vi "Cal Mic Sensitivity.vi"(0 "Device":string) -> (8 "Sens out":dbl)   [LabVIEW 2020]
uses:
  Sub VIs/CalMic-Params.ctl
  <vilib>/DAQmx/read.llb/DAQmx Read (Analog 1D DBL 1Chan NSamp).vi
  <vilib>/Analysis/4window.llb/Hamming Window (DBL).vi
  <vilib>/Analysis/5stat.llb/RMS (DBL).vi
  26d49422-8282-4cac-89f2-fadff3ad3e6e.vi
  d476ff2c-f51a-459e-9784-94b5c1fe9eba.vi
  15152fcf-90b8-4f6a-bf53-2f36ac7739d4.vi
  35692ca8-84b5-411b-8b71-ad00e1a5d34d.vi
  c40c26ba-0181-4530-a77b-ff5f65ea09db.vi
  05361e6f-4f95-456f-9b20-3cc06ed979b3.vi
  d7286415-6cbf-4582-be6d-b454bdd6b62e.vi
  bff657e4-377c-489f-b970-c3d29121513a.vi
  4f9c2216-a235-4407-9711-f98c08391440.vi
  <vilib>/Analysis/baseanly.llb/Mean.vi
  <vilib>/Analysis/baseanly.llb/Mean (DBL).vi
  <vilib>/Analysis/4window.llb/AllCosWindow (DBL).vi
  <vilib>/DAQmx/miscellaneous.llb/DAQmx Fill In Error Info.vi
  epl-vi-lib/Utility VIs/Math VIs/FFT x(t) to dB,Degrees (1D).vi
  <vilib>/Analysis/NI_AALPro.lvlib
  epl-vi-lib/PXI DAQ VIs/TDT VIs/TDT-Signal Bank Action.ctl
panel:
  in  "mV/Pa":dbl=-inf caption="Mic Sens (mV/Pa)"
  in  "Mic Sens (dB V/SPL) in":dbl=-inf
  in  "START":bool
  in  "Sens":dbl=-inf caption="Mic Sens (dB V/SPL)"
  in  "Duration (s)":dbl=1.0
  in  "Sampling Rate (Hz)":dbl=20000.0
  in  "Level (dB SPL)":dbl=124.0 caption="Pistonphone Output\n(dB SPL)" format="%.2f"
  in  "Gain (dB)":dbl=2.0
  out "Magnitude Graph":T1(graph)
  out "Waveform Graph":dbl[](graph)
  in  "finished":errorcluster
  out "Calibration Log":string[][](table)
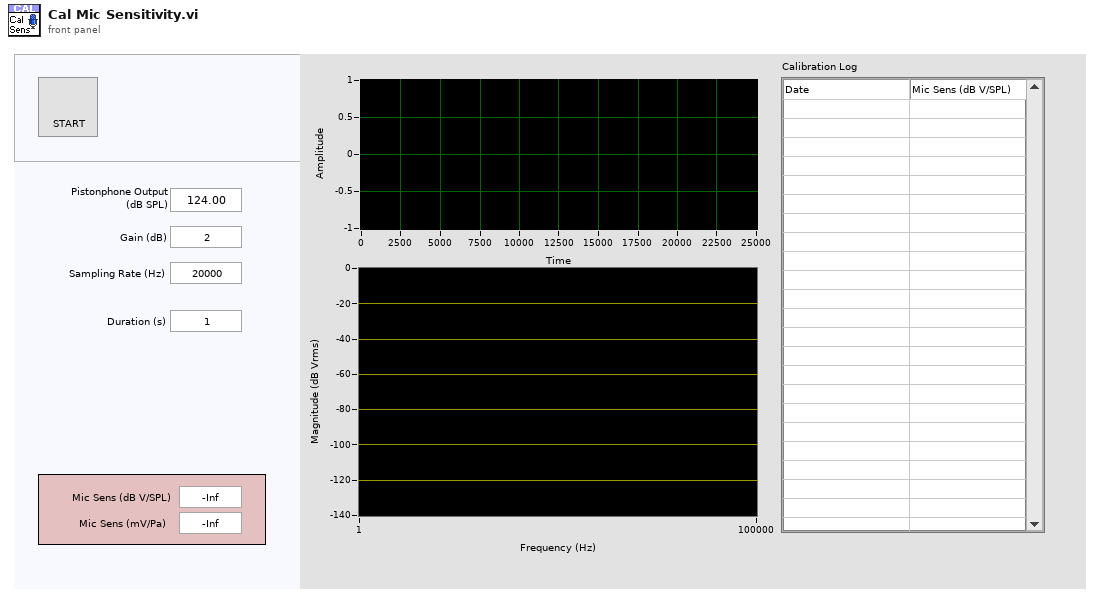
[diagram p1: front panel]
types:
  T1 = cluster{"Freq (Hz)":dbl[], "+Freq. Mag of FFT (dB rms)":dbl[]}
  T2 = typedef "CalMic-Params.ctl" = cluster{"Level (dB SPL)":dbl, "Gain":dbl, "Sampling Rate (Hz)":dbl, "Duration (s)":dbl}
  T3 = cluster{"config":path, "log":path, "acquired":bool}
  T4 = enum8{"Enabled", "Disabled", "Disabled and Grayed Out"}
  T5 = typedef "TDT-Signal Bank Action.ctl" = enum16{"Init", "Write", "Read", "Rewrite", "Reset", "Recycle", "Ramp up", "Ramp down", "Zero"}
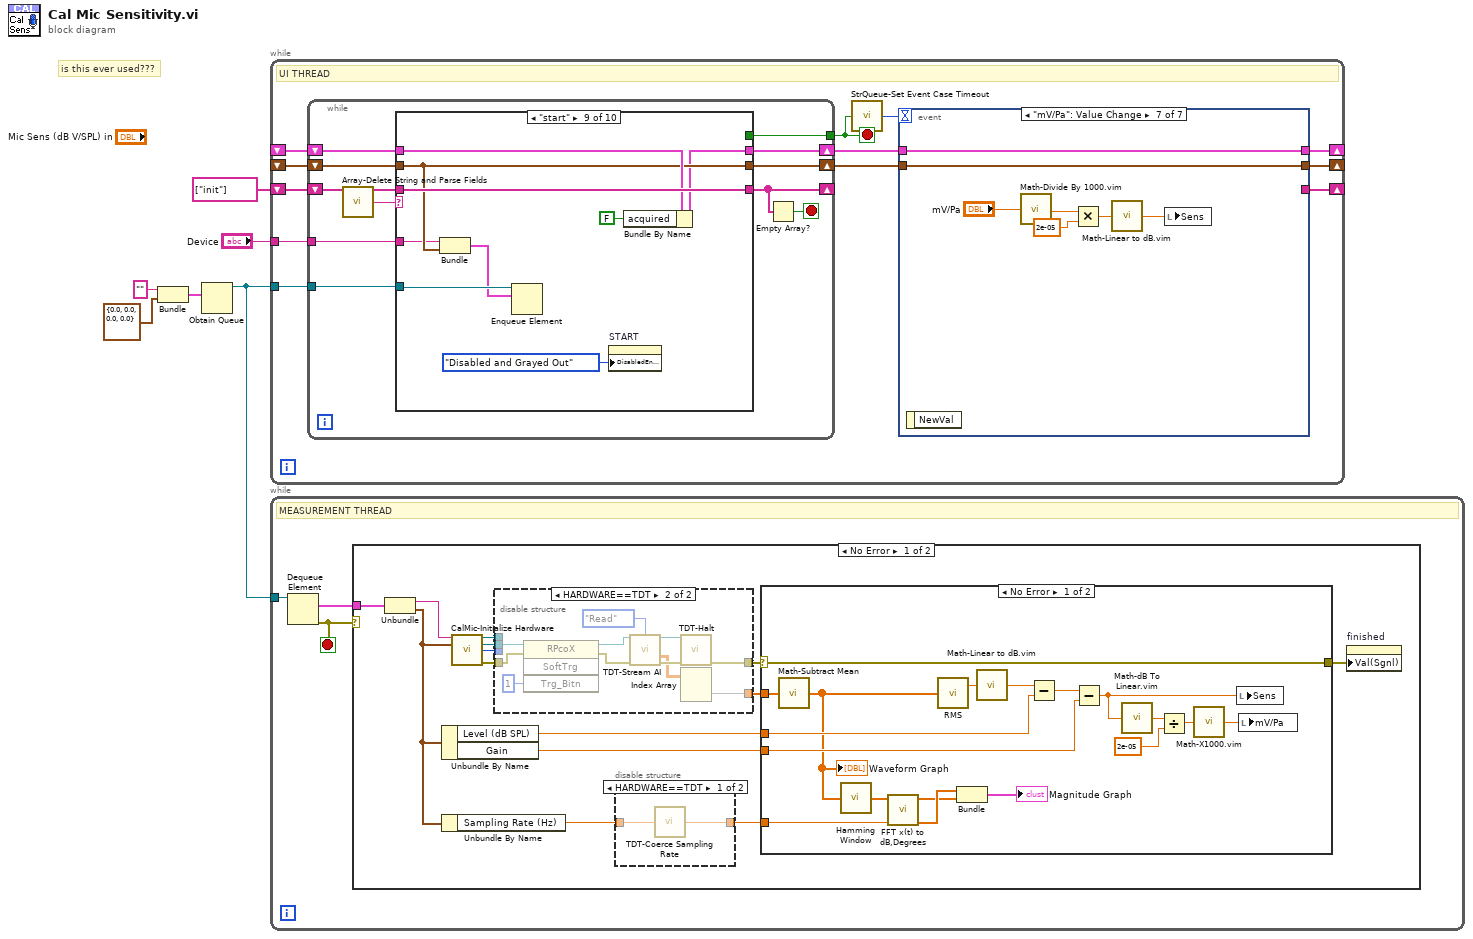
[diagram p0: block diagram]
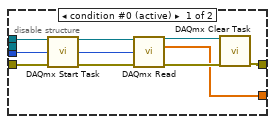
[diagram p3: hidden frame]
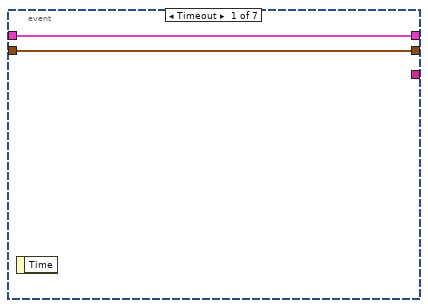
[diagram p6: hidden frame]
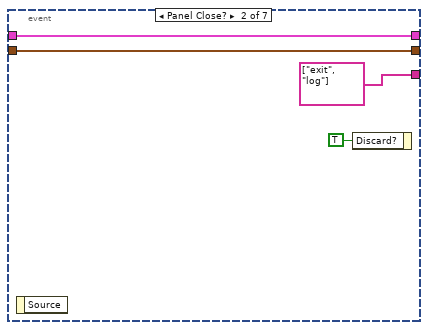
[diagram p7: hidden frame]
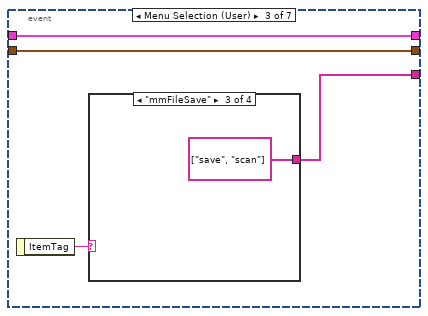
[diagram p8: hidden frame]
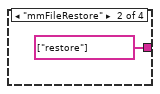
[diagram p10: hidden frame]
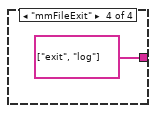
[diagram p11: hidden frame]
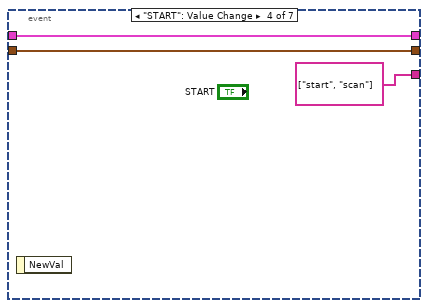
[diagram p12: hidden frame]
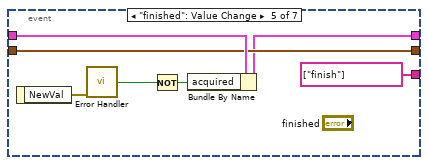
[diagram p13: hidden frame]
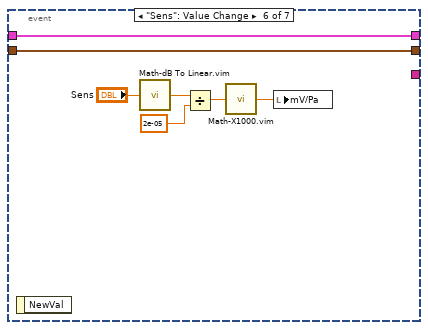
[diagram p14: hidden frame]
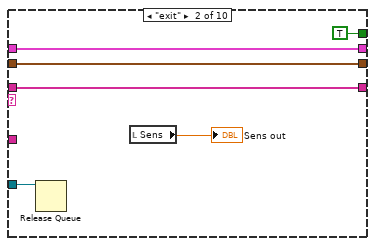
[diagram p16: hidden frame]
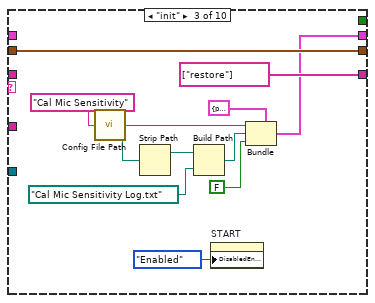
[diagram p17: hidden frame]
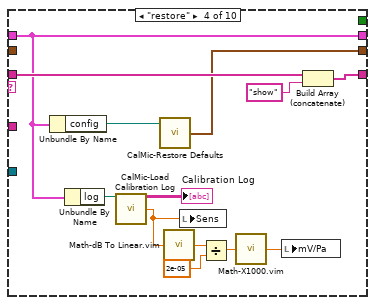
[diagram p18: hidden frame]
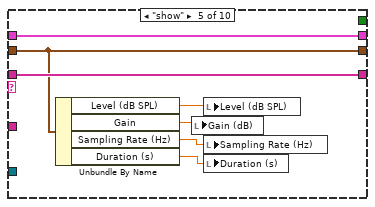
[diagram p19: hidden frame]
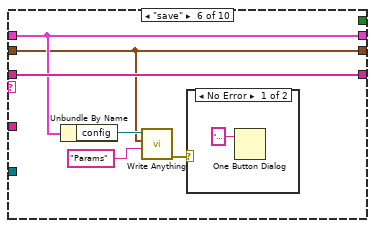
[diagram p20: hidden frame]
diagram:
  # "is this ever used???"
  n1 = Bundle("", "Params"=T2 {"Level (dB SPL)"=0.0, "Gain"=0.0, "Sampling Rate (Hz)"=0.0, "Duration (s)"=0.0}) -> (w2:cluster{string, "Params":T2})  [unwired: 1 in]
  n2 = Obtain Queue(element data type=w2) -> (queue out=w6:refnum<queue>)  [unwired: 4 in, 2 out]
  n3 = while {
    tunnel: w6 -> [w15]
    shift-right: [w14] -> _
    shift-left: string[] ["init"] -> [w18]
    tunnel: "Device" -> [w13]
    shift-right: [w11] -> _
    shift-left: _ -> [w12]
    shift-right: [w8] -> _
    shift-left: _ -> [w7]
    stop <- w17 stop-if-true
    # "UI THREAD"
    n4 = while {
      shift-right: [w67] -> _
      shift-left: w18 -> [w64]
      tunnel: [w65] -> w17
      tunnel: w15 -> [w61]
      tunnel: w13 -> [w60]
      shift-right: [w58] -> w10
      shift-left: w12 -> [w59]
      shift-right: [w57] -> w9
      shift-left: w7 -> [w56]
      stop <- w66 stop-if-true
      n5 = call "Array-Delete String and Parse Fields.vi"("Array in"=w64) -> ("Array out"=w63:string[], "Field 1"=w62:string)  [unwired: 10 in, 3 out]
      n6 = case shown="\"start\"" w62 {
        tunnel: w63 -> [w70 w76 _ w100 w107 w113 w123 w128 w142 w146]
        tunnel: [w70 w76 string[] ["restore"] ("Array out") w98 w107 w113 w123 w128 w142 w146] -> w67
        tunnel: [_ TRUE _ _ _ _ _ _ _ _] -> w65
        tunnel: w61 -> [_ w74 _ _ _ _ _ _ w138 _]
        tunnel: w60 -> [_ _ _ _ _ _ _ _ w134 _]
        tunnel: w59 -> [w69 w73 _ w94 w106 w112 w122 w126 w140 w144]
        tunnel: [w69 w73 w77 w94 w106 w112 w122 w126 w136 w144] -> w58
        tunnel: [w68 w72 w85 w99 w105 w110 w120 w127 w139 w143] -> w57
        tunnel: w56 -> [w68 w72 w85 _ w105 w110 w121 w127 w139 w143]
        frame "", Default {
        }
        frame "exit" {
          n7 = Release Queue(queue=w74) -> ()  [unwired: 2 in, 3 out]
          n8 = local read "Sens"() -> (→"Sens out":dbl)
        }
        frame "init" {
          n9 = call "Config File Path.vi"("AppName"="Cal Mic Sensitivity") -> ("Default config file name"=w80:path)
          n10 = Strip Path(path=w80) -> (stripped path=w83:path)  [unwired: 1 out]
          n11 = Build Path(base path=w83, name or relative path=path "Cal Mic Sensitivity Log.txt") -> (appended path=w79:path)
          n12 = property on="START" class="Bool"("DisabledEnum"=T4."Enabled" ("Disabled")) -> ()  [unwired: 2 in, 2 out]
          n13 = Bundle(cluster=T3 {"config"=path "", "log"=path "", "acquired"=FALSE}, "config"=w80, "log"=w79, "acquired"=FALSE) -> (w77:T3)
        }
        frame "restore" {
          n14 = Unbundle By Name(w94) -> ("config"=w95:path)
          n15 = Unbundle By Name(w94) -> ("log"=w93:path)
          n16 = call "CalMic-Load Calibration Log.vi"("Cal Log"=w93) -> ("Array"=→"Calibration Log":string[][], "Last"=w89:dbl)  [unwired: 13 in]
          n17 = call "CalMic-Restore Defaults.vi"("config"=w95) -> ("Params"=w99:T2)  [unwired: 14 in]
          n18 = call "Math-dB To Linear.vim"("dB"=w89) -> ("linear"=w91:dbl)
          n19 = local write "Sens"(w89) -> ()
          n20 = Divide(x=w91, y=2e-05) -> (x/y=w90:dbl)
          n21 = call "Math-X1000.vim"("X"=w90) -> ("1000X"=w88:dbl)
          n22 = local write "mV/Pa"(w88) -> ()
          n23 = Build Array (concatenate)(w100, "show") -> (w98:string[])
        }
        frame "show" {
          n24 = Unbundle By Name(w105) -> ("Level (dB SPL)"=w104:dbl, "Gain"=w103:dbl, "Sampling Rate (Hz)"=w102:dbl, "Duration (s)"=w101:dbl)
          n25 = local write "Gain (dB)"(w103) -> ()
          n26 = local write "Level (dB SPL)"(w104) -> ()
          n27 = local write "Sampling Rate (Hz)"(w102) -> ()
          n28 = local write "Duration (s)"(w101) -> ()
        }
        frame "save" {
          n29 = Unbundle By Name(w112) -> ("config"=w111:path)
          n30 = call "Write Anything.vi"("Section Name (Name of \"Anything\")"="Params" ("Section Name (Name of \"Anything\")"), "Anything"=w110, "Path (dialog)"=w111) -> ("Error Out"=w108:errorcluster)  [unwired: 7 in, 1 out]
          n31 = case shown="No Error" w108 {
            selector: w108 -> [_ w115]
            frame No Error {
              n32 = One Button Dialog(message="Defaults saved.") -> ()  [unwired: 1 in, 1 out]
            }
            frame Error {
              n33 = call "Error Handler.vi"("error in (no error)"=w115) -> ()  [unwired: 12 in, 3 out]
            }
          }
        }
        frame "scan" {
          n34 = Bundle By Name(cluster=w121, "Level (dB SPL)"="Level (dB SPL)", "Gain"="Gain (dB)", "Duration (s)"="Duration (s)", "Sampling Rate (Hz)"="Sampling Rate (Hz)") -> (w120:T2)
        }
        frame "log" {
          n35 = Unbundle By Name(w126) -> ("log"=w125:path, "acquired"=w124:bool)
          n36 = case shown="True" w124 {
            tunnel: w125 -> [_ w130]
            frame False {
            }
            frame True {
              n37 = local read "Sens"() -> (w133:dbl)
              n38 = Format Date/Time String() -> (date/time string=w129:string)  [unwired: 3 in]
              n39 = Format Into String(format string="%s\t%.2f\n", w129, w133) -> (resulting string=w132:string)  [unwired: 2 in, 1 out]
              n40 = call "Append to Text File.vi"("file path"=w130, "text"=w132) -> ()  [unwired: 12 in, 2 out]
            }
          }
        }
        frame "start" {
          n41 = Bundle("Device"=w134, "Params"=w139) -> (w137:cluster{"Device":string, "Params":T2})  [unwired: 1 in]
          n42 = Enqueue Element(queue=w138, element=w137) -> ()  [unwired: 2 in, 3 out]
          n43 = property on="START" class="Bool"("DisabledEnum"=T4."Disabled and Grayed Out" ("Disabled")) -> ()  [unwired: 2 in, 2 out]
          n44 = Bundle By Name(cluster=w140, "acquired"=FALSE) -> (w136:T3)
        }
        frame "finish" {
          n45 = property on="START" class="Bool"("DisabledEnum"=T4."Enabled" ("Disabled")) -> ()  [unwired: 2 in, 2 out]
        }
      }
      n46 = Empty Array?(array=w67) -> (empty?=w66:bool)
    }
    n47 = call "StrQueue-Set Event Case Timeout.vi"("Quit"=w17) -> ("timeout"=w16:i32)  [unwired: 14 in]
    n48 = event shown="[6] \"mV/Pa\": Value Change" {
      selector: _ -> [_ _ _ _ _ _ _]
      dyn-events: _ -> [_ _ _ _ _ _ _]
      timeout: w16 -> [_ _ _ _ _ _ _]
      tunnel: [_ string[] ["exit", "log"] w27 string[] ["start", "scan"] string[] ["finish"] _ _] -> w14
      tunnel: [w20 w22 w26 w33 w37 w48 w55] -> w11
      tunnel: w10 -> [w20 w22 w26 w33 w41 w48 w55]
      tunnel: w9 -> [w19 w21 w25 w32 w40 w47 w54]
      tunnel: [w19 w21 w25 w32 w40 w47 w54] -> w8
      event Timeout {
        n49 = event-data() -> ()  [unwired: 1 in, 1 out]
      }
      event Panel Close? {
        n50 = event-data() -> ()  [unwired: 1 in, 1 out]
        n51 = event-data("Discard?"=TRUE) -> ()  [unwired: 1 in, 1 out]
      }
      event Menu Selection (User) {
        n52 = event-data() -> ("ItemTag"=w28:string)  [unwired: 1 in]
        n53 = case shown="\"mmFileSave\"" w28 {
          tunnel: [_ string[] ["restore"] string[] ["save", "scan"] string[] ["exit", "log"]] -> w27
          frame "", Default {
          }
          frame "mmFileRestore" {
          }
          frame "mmFileSave" {
          }
          frame "mmFileExit" {
          }
        }
      }
      event "START": Value Change {
        n54 = event-data() -> ()  [unwired: 1 in, 1 out]
      }
      event "finished": Value Change {
        n55 = event-data() -> ("NewVal"=w38:errorcluster)  [unwired: 1 in]
        n56 = call "Error Handler.vi"("error in (no error)"=w38) -> ("error?"=w35:bool)  [unwired: 12 in, 2 out]
        n57 = Not(x=w35) -> (.not. x?=w36:bool)
        n58 = Bundle By Name(cluster=w41, "acquired"=w36) -> (w37:T3)
      }
      event "Sens": Value Change {
        n59 = event-data() -> ()  [unwired: 1 in, 1 out]
        n60 = call "Math-dB To Linear.vim"("dB"="Sens") -> ("linear"=w44:dbl)
        n61 = Divide(x=w44, y=2e-05) -> (x/y=w43:dbl)
        n62 = call "Math-X1000.vim"("X"=w43) -> ("1000X"=w42:dbl)
        n63 = local write "mV/Pa"(w42) -> ()
      }
      event "mV/Pa": Value Change {
        n64 = event-data() -> ()  [unwired: 1 in, 1 out]
        n65 = call "Math-Divide By 1000.vim"("X"="mV/Pa") -> ("1000X"=w52:dbl)
        n66 = Multiply(x=w52, y=2e-05) -> (x*y=w53:dbl)
        n67 = call "Math-Linear to dB.vim"("linear"=w53) -> ("dB"=w50:dbl)
        n68 = local write "Sens"(w50) -> ()
      }
    }
  }
  n69 = while {
    tunnel: w6 -> [w148]
    stop <- w149 stop-if-true
    # "MEASUREMENT THREAD"
    n70 = Dequeue Element(queue=w148) -> (element=w147:cluster{string, "Params":T2}, error out=w149:errorcluster)  [unwired: 2 in, 2 out]
    n71 = case shown="No Error" w149 {
      tunnel: w147 -> [w163 _]
      frame No Error {
        n72 = Unbundle(w163) -> (w156:string, "Params"=w157:T2)
        n73 = Unbundle By Name(w157) -> ("Level (dB SPL)"=w160:dbl, "Gain"=w159:dbl)
        n74 = Unbundle By Name(w157) -> ("Sampling Rate (Hz)"=w151:dbl)
        n75 = call "CalMic-Initialize Hardware.vi"("Device"=w156, "Params"=w157) -> ("task out"=w155:refnum<k21>, "RPcoX out"=w152:refnum<k7>, "npts"=w154:i32, "error out"=w153:errorcluster)  [unwired: 10 in]
        n76 = disable-structure shown="HARDWARE==TDT" {
          disable-tunnel: [w171 w182] -> w162
          disable-tunnel: [w170 w184] -> w161
          disable-tunnel: w155 -> [w169 _]
          disable-tunnel: w154 -> [w168 _]
          disable-tunnel: w153 -> [w167 w179]
          disable-tunnel: w152 -> [_ w180]
          frame condition #0 (active) {
            n77 = call <vilib>:"DAQmx Start Task.vi"("task/channels in"=w169, "error in"=w167) -> ("task out"=w175:refnum<k21>, "error out"=w174:errorcluster)  [unwired: 12 in]
            n78 = call-poly <vilib>:"DAQmx Read.vi"("task/channels in"=w175, "number of samples per channel"=w168, "error in"=w174) -> ("task out"=w173:refnum<k21>, "data"=w171:dbl[], "error out"=w172:errorcluster)  [unwired: 10 in]
            n79 = call <vilib>:"DAQmx Clear Task.vi"("task in"=w173, "error in"=w172) -> ("error out"=w170:errorcluster)  [unwired: 13 in]
          }
          frame condition #1 {
            n80 = invoke class="RPcoX" method="SoftTrg"(reference=w180, error in=w179, "Trg_Bitn"=1) -> (reference out=w178:refnum<k7>, error out=w176:errorcluster)  [unwired: 1 in, 2 out]
            n81 = call "TDT-Stream AI.vi"("RPcox"=w178, "Action"=TDT-Signal_Bank_Action."Read", "error in (no error)"=w176) -> ("RPcoX thru"=w181:refnum<k7>, "AI Waveforms"=w183:dbl[][], "error out"=w185:errorcluster)  [unwired: 10 in]
            n82 = call "TDT-Halt.vi"("RPcoX"=w181, "error in (no error)"=w185) -> ("error out"=w184:errorcluster)  [unwired: 13 in]
            n83 = Index Array(array=w183) -> (element=w182:dbl[])  [unwired: 2 in]
          }
        }
        n84 = disable-structure shown="HARDWARE==TDT" {
          disable-tunnel: w151 -> [w165 w166]
          disable-tunnel: [w164 w166] -> w150
          frame condition #0 {
            n85 = call "TDT-Coerce Sampling Rate.vi"("Fs (Hz)"=w165) -> ("Coerced"=w164:dbl)
          }
          frame condition #1 (active) {
          }
        }
        n86 = case shown="No Error" w161 {
          selector: w161 -> [w199 w205]
          tunnel: w162 -> [w190 _]
          tunnel: w160 -> [w201 _]
          tunnel: w159 -> [w200 _]
          tunnel: [w199 w205] -> w158
          tunnel: w150 -> [w189 _]
          frame No Error {
            n87 = call "Math-Subtract Mean.vi"("Y"=w190) -> ("Y - mean(Y)"=w187:dbl[])  [unwired: 4 in]
            "Waveform Graph" <- w187
            n88 = call-poly <vilib>:"Hamming Window.vi"("X"=w187) -> ("Windowed X"=w188:dbl[])  [unwired: 1 out]
            n89 = call-poly "FFT x(t) to dB,Degrees.vi"("Fs (Hz)"=w189, "X"=w188) -> ("Freq (Hz)"=w198:dbl[], "+Freq. Mag of FFT (dB rms)"=w197:dbl[])  [unwired: 7 in, 1 out]
            n90 = call-poly <vilib>:"RMS.vi"("X"=w187) -> ("rms value"=w204:dbl)  [unwired: 1 out]
            n91 = Bundle("Freq (Hz)"=w198, "+Freq. Mag of FFT (dB rms)"=w197) -> (→"Magnitude Graph":T1)  [unwired: 1 in]
            n92 = call "Math-Linear to dB.vim"("linear"=w204) -> ("dB"=w202:dbl)
            n93 = Subtract(x=w202, y=w201) -> (x-y=w203:dbl)
            n94 = Subtract(x=w203, y=w200) -> (x-y=w192:dbl)
            n95 = call "Math-dB To Linear.vim"("dB"=w192) -> ("linear"=w194:dbl)
            n96 = Divide(x=w194, y=2e-05) -> (x/y=w193:dbl)
            n97 = call "Math-X1000.vim"("X"=w193) -> ("1000X"=w191:dbl)
            n98 = local write "Sens"(w192) -> ()
            n99 = local write "mV/Pa"(w191) -> ()
          }
          frame Error {
          }
        }
        n100 = property on="finished" class="Clust (strict)"("Val(Sgnl)"=w158) -> ()  [unwired: 2 in, 2 out]
      }
      frame Error {
      }
    }
  }
